vi "Write Timing Status.vi"(8 "error in (no error)":errorcluster, 10 "timing status":T1 {"prev start time" format="%d us"; "cycle end time" format="%d us"; "cycle start time" format="%d us"; "tx end time" format="%d us"; "tx start time" format="%d us"; "rx end time" format="%d us"; "rx start time" format="%d us"}, 11 "timing status pointer in":refnum<class "Timing Status.lvclass">) -> (0 "error out":errorcluster, 3 "timing status pointer out":refnum<class "Timing Status.lvclass">)   [LabVIEW 2017, in "DSF Core.lvlib" / "Timing Status.lvclass"]
uses:
  Timing Status.lvclass
  C:/Git/DSF/LabVIEW-Memory/Source/Classes/Pointer/Pointer.lvclass
  Timing Status Data.ctl
  LabVIEW-Memory/Source/Classes/Pointer/Pointer.lvclass
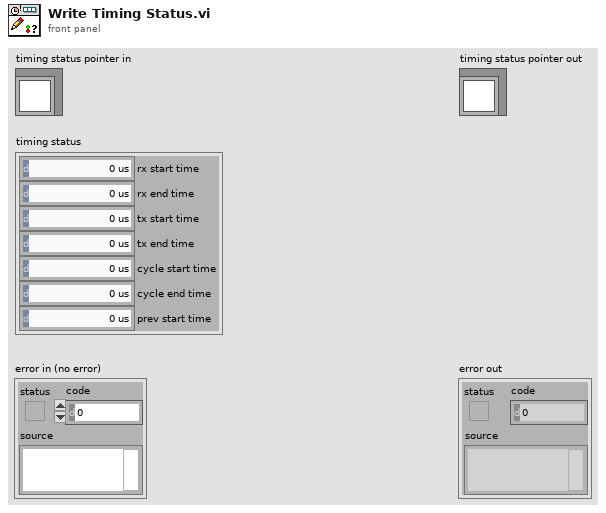
[diagram p1: front panel]
types:
  T1 = typedef "DSF Core.lvlib/Timing Status.lvclass/Timing Status Data.ctl" = cluster{"rx start time":u32, "rx end time":u32, "tx start time":u32, "tx end time":u32, "cycle start time":u32, "cycle end time":u32, "prev start time":u32}
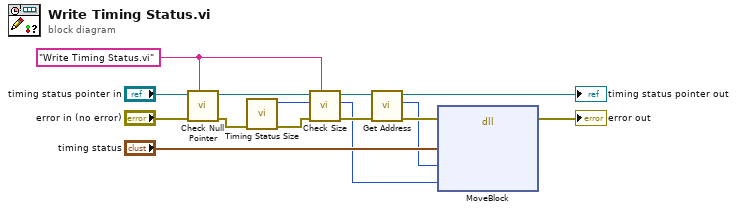
[diagram p0: block diagram]
diagram:
  w3 = "Write Timing Status.vi" ("source vi name")
  n1 = call "Check Null Pointer.vi"("source vi name"=w3, "error in (no error)"="error in (no error)", "Pointer in"="timing status pointer in") -> ("error out"=w2:errorcluster, "Pointer out"=w4:refnum<class "Timing Status.lvclass">)  [unwired: 7 in]
  n2 = call "Timing Status Size.vi"("error in (no error)"=w2) -> ("error out"=w11:errorcluster, "size"=w7:u64)  [unwired: 9 in]
  n3 = call "Check Size.vi"("source vi name"=w3, "error in (no error)"=w11, "required size"=w7, "Pointer in"=w4) -> ("error out"=w13:errorcluster, "required size out"=w6:u64, "Pointer out"=w14:refnum<class "Timing Status.lvclass">)  [unwired: 5 in]
  n4 = call "Get Address.vi"("Pointer in"=w14) -> ("address"=w8:u64, "Pointer out"=→"timing status pointer out":refnum<class "Timing Status.lvclass">)  [unwired: 9 in]
  n5 = dll-call lib="LabVIEW" fn="MoveBlock"(error in=w13, "src"="timing status", "dst"=w8, "size"=w6) -> (error out=→"error out":errorcluster)  [unwired: 6 in, 1 out]
